vi "PH_BeamlineInformation.panel.vi"() -> ()   [LabVIEW 2014, in "PH_BeamlineInformation.lvlib"]
uses:
  PH_BeamlineInformation.lvlib
  PH_Beamline_Chief/PH_Beamline_Chief.Section.ctl
  PH_Basics/PH_SystemInformation/PH_SystemInformation.GUI Refs.ctl
  PH_BeamlineInformation.Powermeter.ctl
  PH_BeamlineInformation.Efficiency.ctl
  PH_BeamlineInformation.GUI Ref.ctl
  PH_Basics/PH_Common/PH_Common.lvlib
  PH_Beamline_Chief/PH_Beamline_Chief.lvlib
  PH_Basics/PH_SystemInformation/PH_SystemInformation.lvlib
  PH_Basics/PH_Class/PH_Class.lvlib
panel:
  in  "Voltage PA 45 DP":dbl caption="[V]"
  in  "Voltage PA 45":dbl caption="[V]"
  in  "Voltage  PA 19-2":dbl caption="[V]"
  in  "Voltage  PA 19-1":dbl caption="[V]"
  in  "Voltage FR":dbl caption="[V]"
  in  "Voltage MA 5":dbl caption="[V]"
  in  "Voltage MA 4":dbl caption="[V]"
  in  "Voltage MA 3":dbl caption="[V]"
  in  "Voltage MA 2":dbl caption="[V]"
  out "PU PA 45 DP":bool caption="State PU"
  in  "Voltage MA 1":dbl caption="[V]"
  out "PU FR":bool caption="State PU"
  out "PU PA 45":bool caption="State PU"
  out "PU PA 19-2":bool caption="State PU"
  out "PU PA 19-1":bool caption="State PU"
  out "PU MA 5":bool caption="State PU"
  out "PU MA 4":bool caption="State PU"
  out "PU MA 3":bool caption="State PU"
  out "PU MA 2":bool caption="State PU"
  out "PU MA 1":bool caption="State PU"
  out "Z6 Comp Losses":dbl=-1.0 format="%#_3g"
  out "Z6_COS_Powermeter_CurrentValue":dbl=-1.0 caption="J"
  out "Z6 green conversion":dbl=-1.0 format="%#_3g"
  out "MA Amplification":dbl=-1.0 format="%#_3g"
  out "PA Amplification":dbl=-1.0 format="%#_3g"
  out "fs_Nearfield_Frontend_ImageOperator_StatisticData":dbl=-1.0 caption="J"
  out "ns_Exit_Powermeter_CurrentValue":dbl=-1.0 caption="J"
  out "Z6_IR_Powermeter_CurrentValue":dbl=-1.0 caption="J"
  out "Z6_green_Powermeter_CurrentValue":dbl=-1.0 caption="J"
  out "PA_Exit_Powermeter_CurrentValue":dbl=-1.0 caption="J"
  out "MAS_Powermeter_CurrentValue":dbl=-1.0 caption="J"
  out "PHELIX_Beamline_MA_LB_BL_Status 2":u32(colorbox)
  out "PHELIX_Beamline_PA_before_Bypass_BL_Status":u32(colorbox)
  out "PHELIX_Beamline_PA_BL_Status":u32(colorbox)
  out "PHELIX_Beamline_LB_TB2_BL_Status":u32(colorbox)
  out "PHELIX_Beamline_Z6_BL_Status":u32(colorbox)
  out "PHELIX_Beamline_LL_BL_Status":u32(colorbox)
  out "PHELIX_Beamline_MA_Exit_BL_Status":u32(colorbox)
  out "PHELIX_Beamline_PA_Exit_BL_Status":u32(colorbox)
  out "PHELIX_Beamline_PA_Input_BL_Status":u32(colorbox)
  out "PHELIX_Beamline_PA_UnDelay_BL_Status":u32(colorbox)
  out "PHELIX_Beamline_fs_YLF_BL_Status":u32(colorbox)
  out "PHELIX_Beamline_YLF_BL_Status 2":u32(colorbox)
  out "PHELIX_Beamline_ns_BL_Status 2":u32(colorbox)
  out "PHELIX_Beamline_PA_Bypass_BL_Status 3":u32(colorbox)
  out "PHELIX_Beamline_PA_Bypass_BL_Status 2":u32(colorbox)
  out "PHELIX_Beamline_PA_Bypass_BL_Status 1":u32(colorbox)
  out "PHELIX_Beamline_PA_Delay_BL_Status 3":u32(colorbox)
  out "PHELIX_Beamline_PA_Delay_BL_Status 1":u32(colorbox)
  out "PHELIX_Beamline_PA_Delay_BL_Status 2":u32(colorbox)
  out "PHELIX_Beamline_MA_Z6_BL_Status":u32(colorbox)
  out "PHELIX_Beamline_MA_LB_BL_Status 1":u32(colorbox)
  out "PHELIX_Beamline_MA_LB_BL_Status":u32(colorbox)
  out "PHELIX_Beamline_YLF_BL_Status 1":u32(colorbox)
  out "PHELIX_Beamline_fs_BL_Status":u32(colorbox)
  out "PHELIX_Beamline_ns_BL_Status 1":u32(colorbox)
  out "PHELIX_Beamline_PA_LL_BL_Status 2":u32(colorbox)
  out "PHELIX_Beamline_PA_LL_BL_Status 1":u32(colorbox)
  out "PHELIX_Beamline_PA_MA_BL_Status":u32(colorbox)
  out "PHELIX_Timing_Mode":enum32{"10 Hz", "0.5 Hz", "Shot"}(radio) caption="Modeselector"
  in  "Delete":bool
  out "PIL_Exp4_ShutterDisabled":u32(colorbox) caption="Z6 enabled"
  out "PIL_Exp1_ShutterDisabled":u32(colorbox) caption="Exp 1 enabled"
  out "PIL_Exp2_ShutterDisabled":u32(colorbox) caption="Exp 2 enabled"
  out "PIL_Exp3_ShutterDisabled":u32(colorbox) caption="Exp 3 enabled"
  out "PIL_disabled_mainamp":u32(colorbox) caption="MA enabled"
  out "PIL_NA_Chain":u32(colorbox) caption="Emergency off"
  out "PIL_disabled_laser":u32(colorbox) caption="Laser enabled"
  out "PIL_disabled_preamp":u32(colorbox) caption="PA enabled"
  out "error out":errorcluster
  in  "error in (no error)":errorcluster
  in  "object ref":refnum<vi>
  out "PHELIX_Beamline_LB_TB3_BL_Status":u32(colorbox)
  # "PCS"
  # "3.40"
  # "Z6"
  # "MA"
  # "ns-FE"
  # "fs-FE"
  # "YLF"
  # "Exp LB"
  # "LL"
  # "PA"
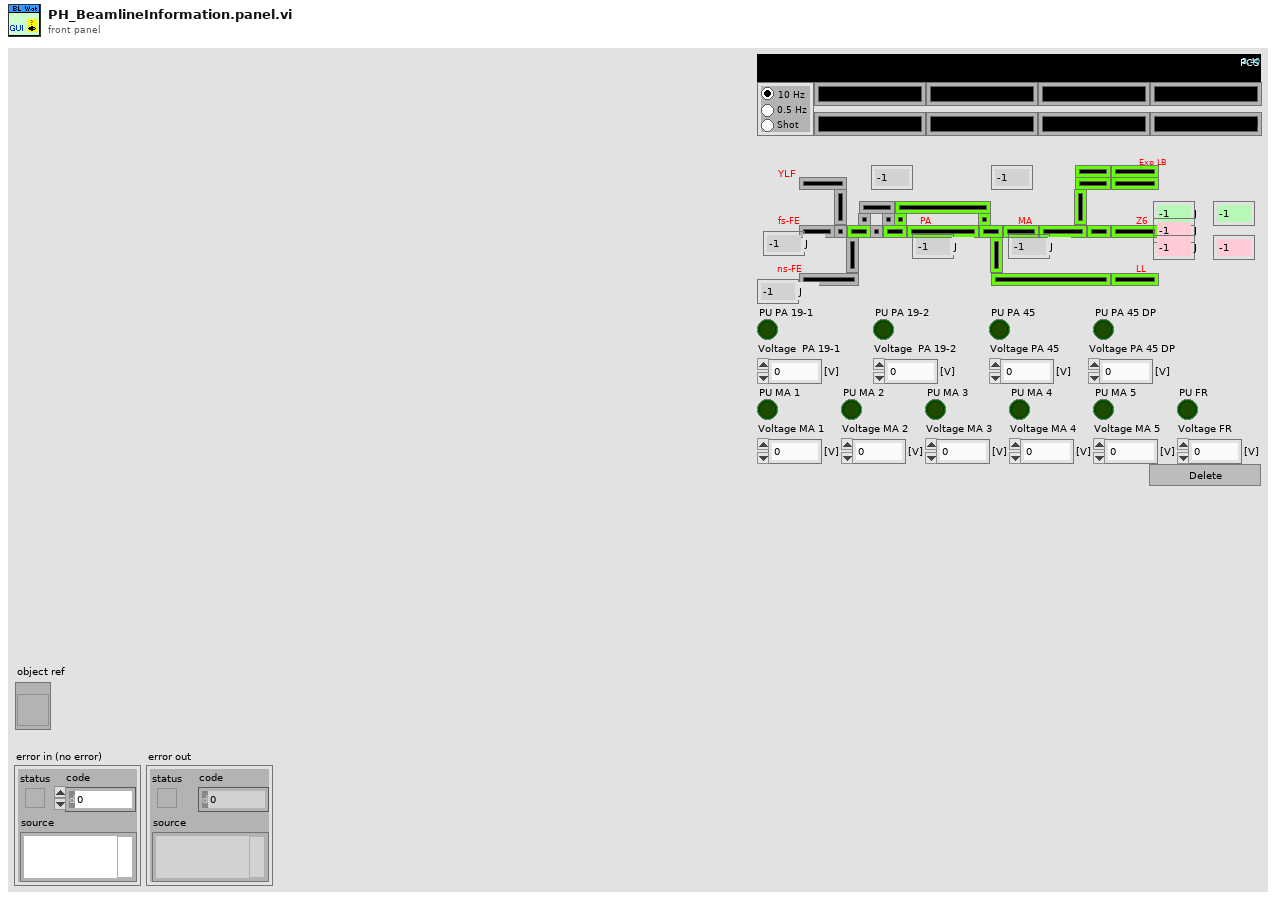
[diagram p1: front panel]
types:
  T1 = typedef "PH_BeamlineInformation.lvlib/PH_BeamlineInformation.GUI Ref.ctl" = cluster{"BL Elements":cluster{"GUI Ref":refnum<vi>, "Beamline Section":T2}[], "Powermeters":T3, "Efficiency GUI Refs":T4, "Head GUI Refs":cluster{"PA - 19 - 1":cluster{"in Use":refnum<vi>, "voltage":refnum<vi>}, "PA - 19 - 2":cluster{"in Use":refnum<vi>, "voltage":refnum<vi>}, "PA - 45":cluster{"in Use":refnum<vi>, "voltage":refnum<vi>}, "PA - 45 - DP":cluster{"in Use":refnum<vi>, "voltage":refnum<vi>}, "MA - 1":cluster{"in Use":refnum<vi>, "voltage":refnum<vi>}, "MA - 2":cluster{"in Use":refnum<vi>, "voltage":refnum<vi>}, "MA - 3":cluster{"in Use":refnum<vi>, "voltage":refnum<vi>}, "MA - 4":cluster{"in Use":refnum<vi>, "voltage":refnum<vi>}, "MA - 5":cluster{"in Use":refnum<vi>, "voltage":refnum<vi>}, "MA - FR":cluster{"in Use":refnum<vi>, "voltage":refnum<vi>}}, "System Information GUI Refs":T5}
  T2 = typedef "PH_Beamline_Chief.lvlib/PH_Beamline_Chief.Section.ctl" = enum16{"None", "YLF", "fs", "fs-YLF", "ns", "PA-Input", "PA-Undelay", "PA-Delay", "PA-before-Bypass", "PA", "PA-Bypass", "PA-Exit", "PA-LL", "LL", "PA-MA", "MA-Exit", "MA-Z6", "Z6", "MA-LB", "LB-TB2", "LB-TB3"}
  T3 = typedef "PH_BeamlineInformation.lvlib/PH_BeamlineInformation.Powermeter.ctl" = cluster{"ns FE":cluster{"GUI Ref":refnum<vi>, "Value":dbl}, "fs FE":cluster{"GUI Ref":refnum<vi>, "Value":dbl}, "PA":cluster{"GUI Ref":refnum<vi>, "Value":dbl}, "MA":cluster{"GUI Ref":refnum<vi>, "Value":dbl}, "Z6 green":cluster{"GUI Ref":refnum<vi>, "Value":dbl}, "Z6 IR":cluster{"GUI Ref":refnum<vi>, "Value":dbl}, "Z6 COS":cluster{"GUI Ref":refnum<vi>, "Value":dbl}}
  T4 = typedef "PH_BeamlineInformation.lvlib/PH_BeamlineInformation.Efficiency.ctl" = cluster{"PA Gain":cluster{"GUI Ref":refnum<vi>, "Value":dbl}, "MA Gain":cluster{"GUI Ref":refnum<vi>, "Value":dbl}, "Z6 green Conversion":cluster{"GUI Ref":refnum<vi>, "Value":dbl}, "Z6 Comp Losses":cluster{"GUI Ref":refnum<vi>, "Value":dbl}}
  T5 = typedef "PH_SystemInformation.lvlib/PH_SystemInformation.GUI Refs.ctl" = cluster{"Laser":refnum<vi>, "PreAmp":refnum<vi>, "MainAmp":refnum<vi>, "Emergency Off":refnum<vi>, "Exp 1":refnum<vi>, "Exp 2":refnum<vi>, "Exp 3":refnum<vi>, "Exp 4":refnum<vi>, "Timing Mode GUI Ref":refnum<vi>}
  T6 = cluster{"PA - 19 - 1":cluster{"in Use":refnum<vi>, "voltage":refnum<vi>}, "PA - 19 - 2":cluster{"in Use":refnum<vi>, "voltage":refnum<vi>}, "PA - 45":cluster{"in Use":refnum<vi>, "voltage":refnum<vi>}, "PA - 45 - DP":cluster{"in Use":refnum<vi>, "voltage":refnum<vi>}, "MA - 1":cluster{"in Use":refnum<vi>, "voltage":refnum<vi>}, "MA - 2":cluster{"in Use":refnum<vi>, "voltage":refnum<vi>}, "MA - 3":cluster{"in Use":refnum<vi>, "voltage":refnum<vi>}, "MA - 4":cluster{"in Use":refnum<vi>, "voltage":refnum<vi>}, "MA - 5":cluster{"in Use":refnum<vi>, "voltage":refnum<vi>}, "MA - FR":cluster{"in Use":refnum<vi>, "voltage":refnum<vi>}}
  T7 = cluster{"GUI Ref":refnum<vi>, "Beamline Section":T2}
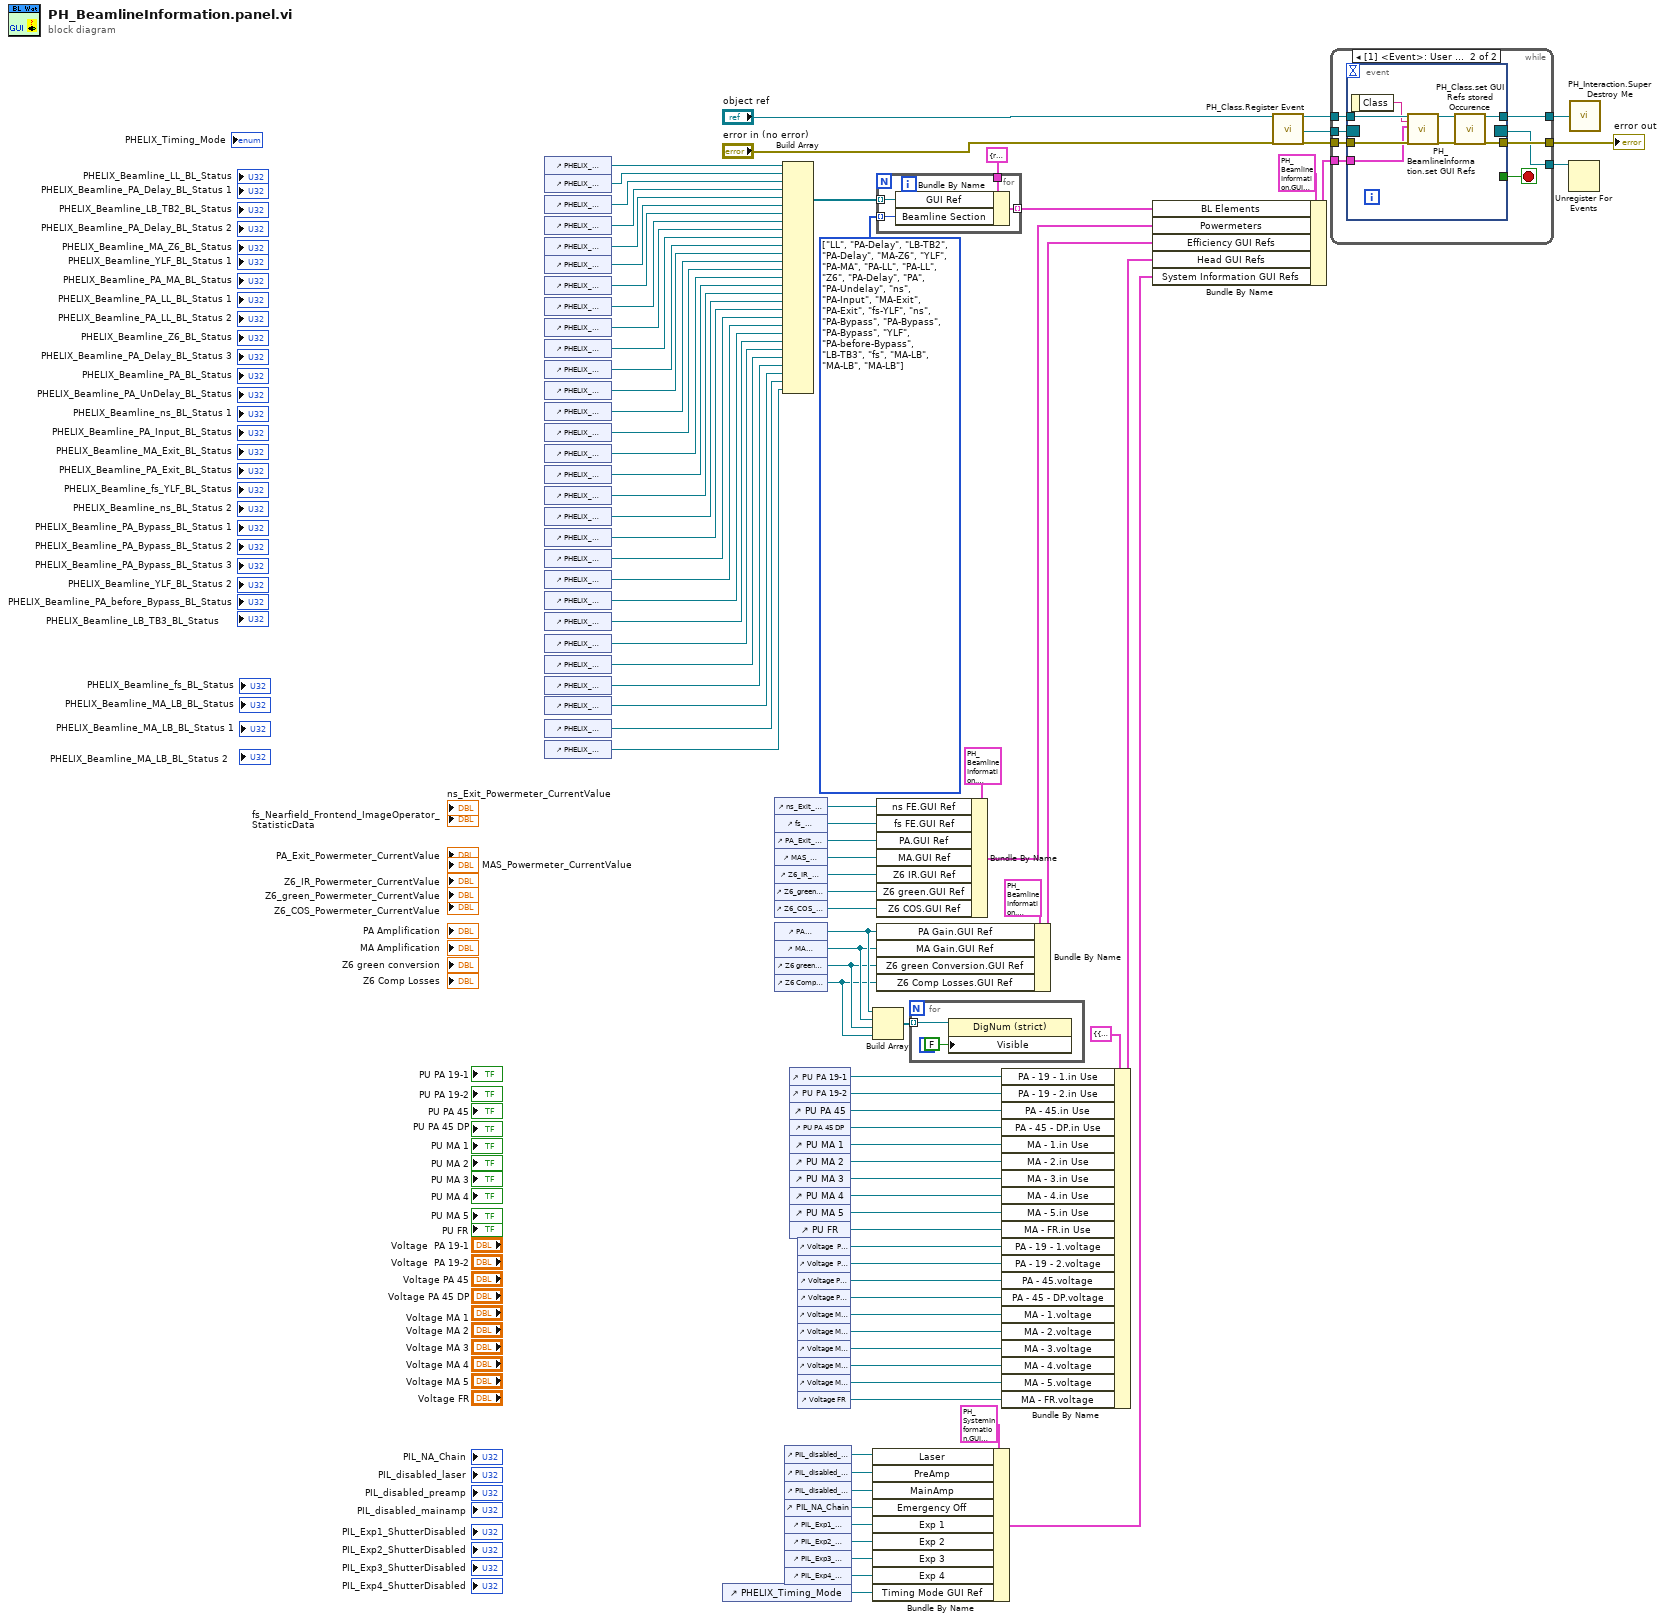
[diagram p0: block diagram]
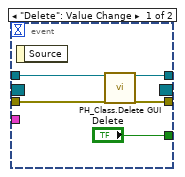
[diagram p2: hidden frame]
diagram:
  w50 = T2[] [enum."LL", enum."PA-Delay", enum."LB-TB2", enum."PA-Delay", enum."MA-Z6", enum."YLF", enum."PA-MA", enum."PA-LL", enum."PA-LL", enum."Z6", enum."PA-Delay", enum."PA", enum."PA-Undelay", enum."ns", enum."PA-Input", enum."MA-Exit", enum."PA-Exit", enum."fs-YLF", enum."ns", enum."PA-Bypass", enum."PA-Bypass", enum."PA-Bypass", enum."YLF", enum."PA-before-Bypass", enum."LB-TB3", enum."fs", enum."MA-LB", enum."MA-LB", enum."MA-LB"] items=["None", "YLF", "fs", "fs-YLF", "ns", "PA-Input", "PA-Undelay", "PA-Delay", "PA-before-Bypass", "PA", "PA-Bypass", "PA-Exit", "PA-LL", "LL", "PA-MA", "MA-Exit", "MA-Z6", "Z6", "MA-LB", "LB-TB2", "LB-TB3"]
  n1 = control-ref of="PHELIX_Beamline_LL_BL_Status"() -> (w90:refnum<vi>)
  n2 = control-ref of="PHELIX_Beamline_PA_Delay_BL_Status 1"() -> (w89:refnum<vi>)
  n3 = control-ref of="PHELIX_Beamline_LB_TB2_BL_Status"() -> (w88:refnum<vi>)
  n4 = control-ref of="PHELIX_Beamline_PA_Delay_BL_Status 2"() -> (w87:refnum<vi>)
  n5 = control-ref of="PHELIX_Beamline_MA_Z6_BL_Status"() -> (w86:refnum<vi>)
  n6 = control-ref of="PHELIX_Beamline_YLF_BL_Status 1"() -> (w85:refnum<vi>)
  n7 = control-ref of="PHELIX_Beamline_PA_MA_BL_Status"() -> (w84:refnum<vi>)
  n8 = control-ref of="PHELIX_Beamline_PA_LL_BL_Status 1"() -> (w83:refnum<vi>)
  n9 = control-ref of="PHELIX_Beamline_PA_LL_BL_Status 2"() -> (w82:refnum<vi>)
  n10 = control-ref of="PHELIX_Beamline_Z6_BL_Status"() -> (w81:refnum<vi>)
  n11 = control-ref of="PHELIX_Beamline_PA_Delay_BL_Status 3"() -> (w80:refnum<vi>)
  n12 = control-ref of="PHELIX_Beamline_PA_BL_Status"() -> (w79:refnum<vi>)
  n13 = control-ref of="PHELIX_Beamline_PA_UnDelay_BL_Status"() -> (w78:refnum<vi>)
  n14 = control-ref of="PHELIX_Beamline_ns_BL_Status 1"() -> (w77:refnum<vi>)
  n15 = control-ref of="PHELIX_Beamline_PA_Input_BL_Status"() -> (w76:refnum<vi>)
  n16 = control-ref of="PHELIX_Beamline_MA_Exit_BL_Status"() -> (w75:refnum<vi>)
  n17 = control-ref of="PHELIX_Beamline_PA_Exit_BL_Status"() -> (w74:refnum<vi>)
  n18 = control-ref of="PHELIX_Beamline_fs_YLF_BL_Status"() -> (w73:refnum<vi>)
  n19 = control-ref of="PHELIX_Beamline_ns_BL_Status 2"() -> (w72:refnum<vi>)
  n20 = control-ref of="PHELIX_Beamline_PA_Bypass_BL_Status 1"() -> (w71:refnum<vi>)
  n21 = control-ref of="PHELIX_Beamline_PA_Bypass_BL_Status 2"() -> (w70:refnum<vi>)
  n22 = control-ref of="PHELIX_Beamline_PA_Bypass_BL_Status 3"() -> (w69:refnum<vi>)
  n23 = control-ref of="PHELIX_Beamline_YLF_BL_Status 2"() -> (w68:refnum<vi>)
  n24 = control-ref of="PHELIX_Beamline_PA_before_Bypass_BL_Status"() -> (w67:refnum<vi>)
  n25 = control-ref of="PHELIX_Beamline_LB_TB3_BL_Status"() -> (w57:refnum<vi>)
  n26 = control-ref of="PHELIX_Beamline_fs_BL_Status"() -> (w56:refnum<vi>)
  n27 = control-ref of="PHELIX_Beamline_MA_LB_BL_Status"() -> (w55:refnum<vi>)
  n28 = control-ref of="PHELIX_Beamline_MA_LB_BL_Status 1"() -> (w54:refnum<vi>)
  n29 = control-ref of="PHELIX_Beamline_MA_LB_BL_Status 2"() -> (w53:refnum<vi>)
  n30 = control-ref of="PHELIX_Timing_Mode"() -> (w14:refnum<vi>)
  n31 = control-ref of="ns_Exit_Powermeter_CurrentValue"() -> (w46:refnum<vi>)
  n32 = control-ref of="fs_Nearfield_Frontend_ImageOperator_StatisticData"() -> (w47:refnum<vi>)
  n33 = control-ref of="PA_Exit_Powermeter_CurrentValue"() -> (w45:refnum<vi>)
  n34 = control-ref of="MAS_Powermeter_CurrentValue"() -> (w43:refnum<vi>)
  n35 = control-ref of="Z6_IR_Powermeter_CurrentValue"() -> (w44:refnum<vi>)
  n36 = control-ref of="Z6_green_Powermeter_CurrentValue"() -> (w42:refnum<vi>)
  n37 = control-ref of="Z6_COS_Powermeter_CurrentValue"() -> (w41:refnum<vi>)
  n38 = control-ref of="PA Amplification"() -> (w40:refnum<vi>)
  n39 = control-ref of="MA Amplification"() -> (w39:refnum<vi>)
  n40 = control-ref of="Z6 green conversion"() -> (w38:refnum<vi>)
  n41 = control-ref of="Z6 Comp Losses"() -> (w37:refnum<vi>)
  n42 = Build Array(w90, w89, w88, w87, w86, w85, w84, w83, w82, w81, w80, w79, w78, w77, w76, w75, w74, w73, w72, w71, w70, w69, w68, w67, w57, w56, w55, w54, w53) -> (w51:refnum<vi>[])
  n43 = control-ref of="PIL_disabled_laser"() -> (w65:refnum<vi>)
  n44 = control-ref of="PIL_disabled_preamp"() -> (w64:refnum<vi>)
  n45 = control-ref of="PIL_disabled_mainamp"() -> (w63:refnum<vi>)
  n46 = control-ref of="PIL_NA_Chain"() -> (w62:refnum<vi>)
  n47 = control-ref of="PIL_Exp1_ShutterDisabled"() -> (w61:refnum<vi>)
  n48 = control-ref of="PIL_Exp2_ShutterDisabled"() -> (w60:refnum<vi>)
  n49 = control-ref of="PIL_Exp3_ShutterDisabled"() -> (w59:refnum<vi>)
  n50 = control-ref of="PIL_Exp4_ShutterDisabled"() -> (w58:refnum<vi>)
  n51 = control-ref of="PU PA 19-1"() -> (w35:refnum<vi>)
  n52 = control-ref of="PU PA 19-2"() -> (w34:refnum<vi>)
  n53 = control-ref of="PU PA 45"() -> (w33:refnum<vi>)
  n54 = control-ref of="PU PA 45 DP"() -> (w26:refnum<vi>)
  n55 = control-ref of="PU MA 1"() -> (w31:refnum<vi>)
  n56 = control-ref of="PU MA 2"() -> (w30:refnum<vi>)
  n57 = control-ref of="PU MA 3"() -> (w29:refnum<vi>)
  n58 = control-ref of="PU MA 4"() -> (w28:refnum<vi>)
  n59 = control-ref of="PU MA 5"() -> (w27:refnum<vi>)
  n60 = control-ref of="PU FR"() -> (w25:refnum<vi>)
  n61 = control-ref of="Voltage  PA 19-1"() -> (w24:refnum<vi>)
  n62 = control-ref of="Voltage  PA 19-2"() -> (w23:refnum<vi>)
  n63 = control-ref of="Voltage PA 45"() -> (w22:refnum<vi>)
  n64 = control-ref of="Voltage PA 45 DP"() -> (w21:refnum<vi>)
  n65 = control-ref of="Voltage MA 1"() -> (w20:refnum<vi>)
  n66 = control-ref of="Voltage MA 2"() -> (w19:refnum<vi>)
  n67 = control-ref of="Voltage MA 3"() -> (w18:refnum<vi>)
  n68 = control-ref of="Voltage MA 4"() -> (w17:refnum<vi>)
  n69 = control-ref of="Voltage MA 5"() -> (w16:refnum<vi>)
  n70 = control-ref of="Voltage FR"() -> (w15:refnum<vi>)
  n71 = Build Array(w40, w39, w38, w37) -> (w36:refnum<vi>[])
  n72 = Bundle By Name(cluster=T5 {"Laser"=refnum, "PreAmp"=refnum, "MainAmp"=refnum, "Emergency Off"=refnum, "Exp 1"=refnum, "Exp 2"=refnum, "Exp 3"=refnum, "Exp 4"=refnum, "Timing Mode GUI Ref"=refnum} ("7Color GUI Refs"), "Laser"=w65, "PreAmp"=w64, "MainAmp"=w63, "Emergency Off"=w62, "Exp 1"=w61, "Exp 2"=w60, "Exp 3"=w59, "Exp 4"=w58, "Timing Mode GUI Ref"=w14) -> (w2:T5)
  n73 = for {
    tunnel: T7 {"GUI Ref"=refnum, "Beamline Section"=enum."None"} ("BL Element") -> [w96]
    tunnel: [w95] -> w8 mode=indexing
    tunnel: w51 -> [w94] mode=indexing
    tunnel: w50 -> [w93] mode=indexing
    n74 = Bundle By Name(cluster=w96, "GUI Ref"=w94, "Beamline Section"=w93) -> (w95:T7)
  }
  n75 = Bundle By Name(cluster=T3 {"ns FE"={"GUI Ref"=refnum, "Value"=-1.0}, "fs FE"={"GUI Ref"=refnum, "Value"=-1.0}, "PA"={"GUI Ref"=refnum, "Value"=-1.0}, "MA"={"GUI Ref"=refnum, "Value"=-1.0}, "Z6 green"={"GUI Ref"=refnum, "Value"=-1.0}, "Z6 IR"={"GUI Ref"=refnum, "Value"=-1.0}, "Z6 COS"={"GUI Ref"=refnum, "Value"=-1.0}} ("Powermeters"), "ns FE.GUI Ref"=w46, "fs FE.GUI Ref"=w47, "PA.GUI Ref"=w45, "MA.GUI Ref"=w43, "Z6 IR.GUI Ref"=w44, "Z6 green.GUI Ref"=w42, "Z6 COS.GUI Ref"=w41) -> (w7:T3)
  n76 = Bundle By Name(cluster=T4 {"PA Gain"={"GUI Ref"=refnum, "Value"=-1.0}, "MA Gain"={"GUI Ref"=refnum, "Value"=-1.0}, "Z6 green Conversion"={"GUI Ref"=refnum, "Value"=-1.0}, "Z6 Comp Losses"={"GUI Ref"=refnum, "Value"=-1.0}} ("Efficiency GUI Refs"), "PA Gain.GUI Ref"=w40, "MA Gain.GUI Ref"=w39, "Z6 green Conversion.GUI Ref"=w38, "Z6 Comp Losses.GUI Ref"=w37) -> (w6:T4)
  n77 = for {
    tunnel: w36 -> [w98] mode=indexing
    n78 = property class="DigNum (strict)"(reference=w98, "Visible"=FALSE) -> ()  [unwired: 1 in, 2 out]
  }
  n79 = Bundle By Name(cluster=T6 {"PA - 19 - 1"={"in Use"=refnum, "voltage"=refnum}, "PA - 19 - 2"={"in Use"=refnum, "voltage"=refnum}, "PA - 45"={"in Use"=refnum, "voltage"=refnum}, "PA - 45 - DP"={"in Use"=refnum, "voltage"=refnum}, "MA - 1"={"in Use"=refnum, "voltage"=refnum}, "MA - 2"={"in Use"=refnum, "voltage"=refnum}, "MA - 3"={"in Use"=refnum, "voltage"=refnum}, "MA - 4"={"in Use"=refnum, "voltage"=refnum}, "MA - 5"={"in Use"=refnum, "voltage"=refnum}, "MA - FR"={"in Use"=refnum, "voltage"=refnum}} ("Head GUI Refs"), "PA - 19 - 1.in Use"=w35, "PA - 19 - 2.in Use"=w34, "PA - 45.in Use"=w33, "PA - 45 - DP.in Use"=w26, "MA - 1.in Use"=w31, "MA - 2.in Use"=w30, "MA - 3.in Use"=w29, "MA - 4.in Use"=w28, "MA - 5.in Use"=w27, "MA - FR.in Use"=w25, "PA - 19 - 1.voltage"=w24, "PA - 19 - 2.voltage"=w23, "PA - 45.voltage"=w22, "PA - 45 - DP.voltage"=w21, "MA - 1.voltage"=w20, "MA - 2.voltage"=w19, "MA - 3.voltage"=w18, "MA - 4.voltage"=w17, "MA - 5.voltage"=w16, "MA - FR.voltage"=w15) -> (w5:T6)
  n80 = Bundle By Name(cluster=T1 {"BL Elements"=[], "Powermeters"={"ns FE"={"GUI Ref"=refnum, "Value"=-1.0}, "fs FE"={"GUI Ref"=refnum, "Value"=-1.0}, "PA"={"GUI Ref"=refnum, "Value"=-1.0}, "MA"={"GUI Ref"=refnum, "Value"=-1.0}, "Z6 green"={"GUI Ref"=refnum, "Value"=-1.0}, "Z6 IR"={"GUI Ref"=refnum, "Value"=-1.0}, "Z6 COS"={"GUI Ref"=refnum, "Value"=-1.0}}, "Efficiency GUI Refs"={"PA Gain"={"GUI Ref"=refnum, "Value"=-1.0}, "MA Gain"={"GUI Ref"=refnum, "Value"=-1.0}, "Z6 green Conversion"={"GUI Ref"=refnum, "Value"=-1.0}, "Z6 Comp Losses"={"GUI Ref"=refnum, "Value"=-1.0}}, "Head GUI Refs"={"PA - 19 - 1"={"in Use"=refnum, "voltage"=refnum}, "PA - 19 - 2"={"in Use"=refnum, "voltage"=refnum}, "PA - 45"={"in Use"=refnum, "voltage"=refnum}, "PA - 45 - DP"={"in Use"=refnum, "voltage"=refnum}, "MA - 1"={"in Use"=refnum, "voltage"=refnum}, "MA - 2"={"in Use"=refnum, "voltage"=refnum}, "MA - 3"={"in Use"=refnum, "voltage"=refnum}, "MA - 4"={"in Use"=refnum, "voltage"=refnum}, "MA - 5"={"in Use"=refnum, "voltage"=refnum}, "MA - FR"={"in Use"=refnum, "voltage"=refnum}}, "System Information GUI Refs"={"Laser"=refnum, "PreAmp"=refnum, "MainAmp"=refnum, "Emergency Off"=refnum, "Exp 1"=refnum, "Exp 2"=refnum, "Exp 3"=refnum, "Exp 4"=refnum, "Timing Mode GUI Ref"=refnum}} ("BeamlineInformation GUI Refs"), "BL Elements"=w8, "Powermeters"=w7, "Efficiency GUI Refs"=w6, "Head GUI Refs"=w5, "System Information GUI Refs"=w2) -> (w1:T1)
  n81 = call "PH_Class.Register Event.vi"("i ref in"="object ref", "error in (no error)"="error in (no error)") -> ("i ref out"=w13:refnum<vi>, "Event Registration Refnum"=w11:refnum<event-registration>, "error out"=w12:errorcluster)  [unwired: 15 in]
  n82 = while {
    tunnel: w13 -> [w103]
    tunnel: [w102] -> w92
    tunnel: [w105] -> w91
    tunnel: w12 -> [w104]
    tunnel: w11 -> [w101]
    tunnel: [w100] -> w10
    tunnel: w1 -> [w99]
    stop <- w106 stop-if-true
    n83 = event shown="[1] <Event>: User Event" {
      selector: w101 -> [_ _]
      dyn-events: [_ _] -> w100
      timeout: _ -> [_ _]
      tunnel: ["Delete" _] -> w106
      tunnel: w103 -> [w108 w119]
      tunnel: [w109 w114] -> w105
      tunnel: w104 -> [w110 w117]
      tunnel: [w107 w112] -> w102
      tunnel: w99 -> [_ w115]
      event "Delete": Value Change {
        n84 = event-data() -> ()  [unwired: 1 in, 1 out]
        n85 = call "PH_Class.Delete GUI.vi"("VI in"=w108, "error in (no error)"=w110) -> ("VI out"=w107:refnum<vi>, "error out"=w109:errorcluster)  [unwired: 16 in]
      }
      event User Event {
        n86 = event-data() -> ("Class"=w116:string)  [unwired: 1 in]
        n87 = call "PH_BeamlineInformation.set GUI Refs.vi"("Ref in"=w119, "Class"=w116, "BeamlineInformation GUI Refs"=w115, "error in"=w117) -> ("Ref out"=w113:refnum<vi>, "error out"=w118:errorcluster)  [unwired: 14 in]
        n88 = call "PH_Class.set GUI Refs stored Occurence.vi"("i ref in"=w113, "error in (no error)"=w118) -> ("i ref out"=w112:refnum<vi>, "error out"=w114:errorcluster)  [unwired: 16 in]
      }
    }
  }
  "error out" <- w91
  n89 = Unregister For Events(event registration refnum=w10) -> ()  [unwired: 1 in, 1 out]
  n90 = call "PH_Interaction.Super Destroy Me.vi"("i ref out"=w92) -> ()
